vi "Manage Drive.vi"(7 "Min Drive Free Space (%)":dbl, 8 "error in":errorcluster, 11 "Data Folder":path=path "c:/data") -> (0 "error out":errorcluster, 2 "Drive Space Below Limit":bool)   [LabVIEW 2014]
uses:
  Globals/Global - Monitoring Variables.vi
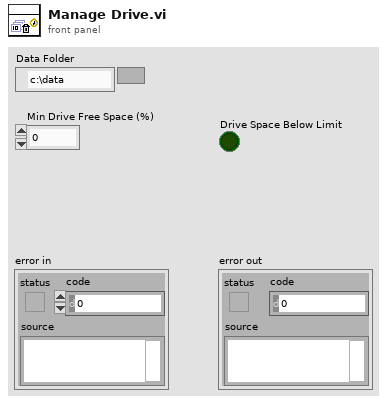
[diagram p1: front panel]
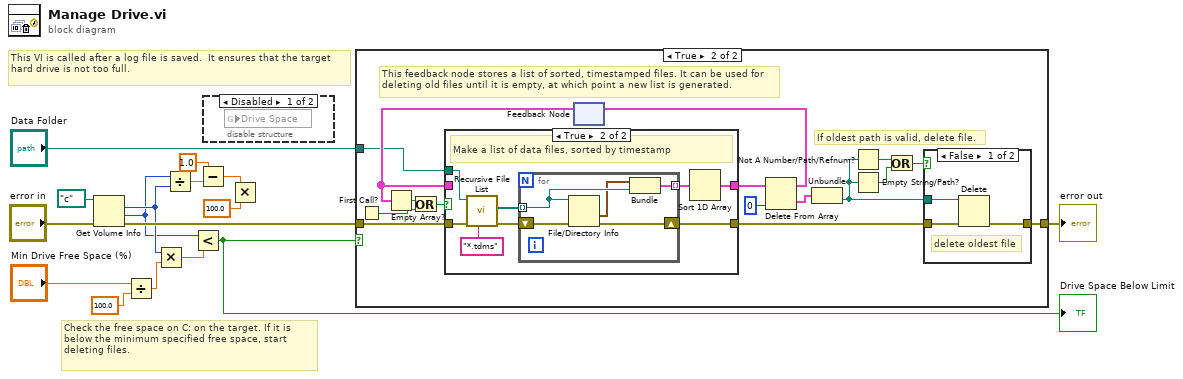
[diagram p0: block diagram]
diagram:
  # "Check the free space on C: on the target. If it is below the minimum specified free space, start deleting files."
  # "This VI is called after a log file is saved.  It ensures that the target hard drive is not too full."
  n1 = Get Volume Info(8:"error in", 11:path "c:/" ("path")) -> (0:w9:errorcluster, 1:w6:i64, 2:w7:i64)  [unwired: 3 out]
  n2 = Divide(x="Min Drive Free Space (%)", y=100.0) -> (x/y=w13:dbl)
  n3 = Multiply(x=w7, y=w13) -> (x*y=w16:dbl)
  n4 = Divide(x=w6, y=w7) -> (x/y=w5:dbl)
  n5 = Less?(x=w6, y=w16) -> (x < y?=w10:bool)
  "Drive Space Below Limit" <- w10
  n6 = Subtract(x=1.0, y=w5) -> (x-y=w3:dbl)
  n7 = disable-structure shown="Disabled" {
    frame Disabled {
      n8 = global read "Global - Monitoring Variables.vi" "Drive Space"() -> ()  [unwired: 1 in]
    }
    frame Enabled {
    }
  }
  n9 = Multiply(x=w3, y=100.0) -> ()  [unwired: 1 out]
  n10 = case shown="True" w10 {
    tunnel: w9 -> [w17 w33]
    tunnel: [w17 w28] -> w8
    tunnel: "Data Folder" -> [_ w24]
    frame False {
      # "Free space is not below the minimum threshold.  Do nothing."
    }
    frame True {
      # "If oldest path is valid, delete file."
      # "This feedback node stores a list of sorted, timestamped files. It can be used for deleting old files until it is empty, at which point a new list is generated."
      n11 = First Call?() -> (First Call?: T/F=w31:bool)
      n12 = feedback #1() -> (w26:cluster{"last mod":timestamp, path}[])  [unwired: 1 out]
      n13 = Empty Array?(array=w26) -> (empty?=w25:bool)
      n14 = Or(x=w25, y=w31) -> (x .or. y?=w32:bool)
      n15 = case shown="True" w32 {
        tunnel: w33 -> [w39 w47]
        tunnel: [w39 w43] -> w27
        tunnel: [w38 w41] -> w30
        tunnel: w26 -> [w38 _]
        tunnel: w24 -> [_ w40]
        frame False {
          # "Current list of old files is non-empty.  Use it."
        }
        frame True {
          # "Make a list of data files, sorted by timestamp"
          n16 = call <vilib>:"Recursive File List.vi"("pattern"="*.tdms", "error in (no error)"=w47, "Folder Path"=w40) -> ("error out"=w44:errorcluster, "All Files in Dir"=w45:path[])  [unwired: 1 in, 6 out]
          n17 = for {
            tunnel: w45 -> [w49] mode=indexing
            shift-right: [w51] -> w43
            shift-left: w44 -> [w52]
            tunnel: [w50] -> w42 mode=indexing
            n18 = File/Directory Info(path=w49, error in=w52) -> (last mod=w48:timestamp, error out=w51:errorcluster)  [unwired: 5 out]
            n19 = Bundle("last mod"=w48, w49) -> (w50:cluster{"last mod":timestamp, path})  [unwired: 1 out]
          }
          n20 = Sort 1D Array(array=w42) -> (sorted array=w41:cluster{"last mod":timestamp, path}[])
        }
      }
      n21 = Delete From Array(array=w30, index=0) -> (deleted portion=w22:cluster{"last mod":timestamp, path}, array with subset deleted=w29:cluster{"last mod":timestamp, path}[])  [unwired: 1 in]
      n22 = feedback-in #1(w29) -> ()
      n23 = Unbundle(w22) -> (w21:path)  [unwired: 1 out]
      n24 = Not A Number/Path/Refnum?(number/path/refnum=w21) -> (NaN/Path/Refnum?=w20:bool)
      n25 = Empty String/Path?(string/path=w21) -> (empty?=w19:bool)
      n26 = Or(x=w20, y=w19) -> (x .or. y?=w18:bool)
      n27 = case shown="False" w18 {
        tunnel: [w36 w37] -> w28
        tunnel: w27 -> [w35 w37]
        tunnel: w21 -> [w34 _]
        frame False {
          # "delete oldest file"
          n28 = Delete(path (use dialog)=w34, error in=w35) -> (error out=w36:errorcluster)  [unwired: 5 out]
        }
        frame True {
        }
      }
    }
  }
  "error out" <- w8
